vi "FTW-Reply-Construct.vi"(5 "Address":string, 11 "error in":errorcluster) -> (4 "FTW-Router Out":refnum<class "FTW-Reply.lvclass">, 6 "Actual Address":string, 10 "Event Registration Refnum":refnum<event-registration>, 15 "error out":errorcluster)   [LabVIEW 2013, in "FTW-Reply.lvclass"]
uses:
  FTW-Reply.lvclass
  Message/Request/FTW-Message-IncomingRequest.lvclass
  Ether/FTW-Ether-EndpointType.ctl
  Endpoint/FTW-Endpoint.lvclass
  FTW-Reply.lvclass/FTW-Reply.ctl
  Ether/FTW-Ether.lvclass
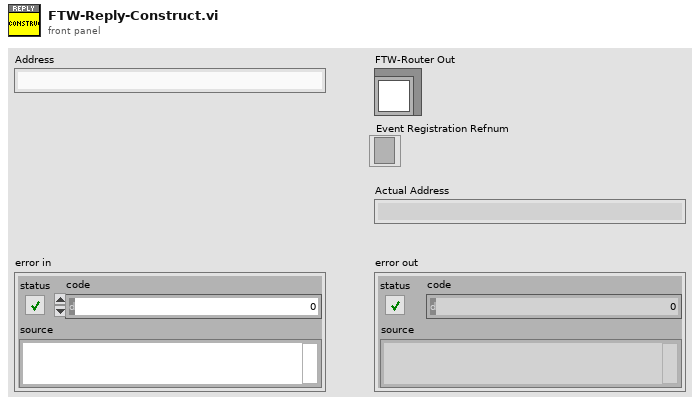
[diagram p1: front panel]
types:
  T1 = typedef "FTW-Ether.lvclass/FTW-Ether-EndpointType.ctl" = enum16{"Server", "Client", "Publisher", "Subscriber"}
  T2 = typedef "FTW-Ether.lvclass/FTW-Ether-MessageTransportScheme.ctl" = enum16{"In process (inproc://)", "TCP (tcp://)"}
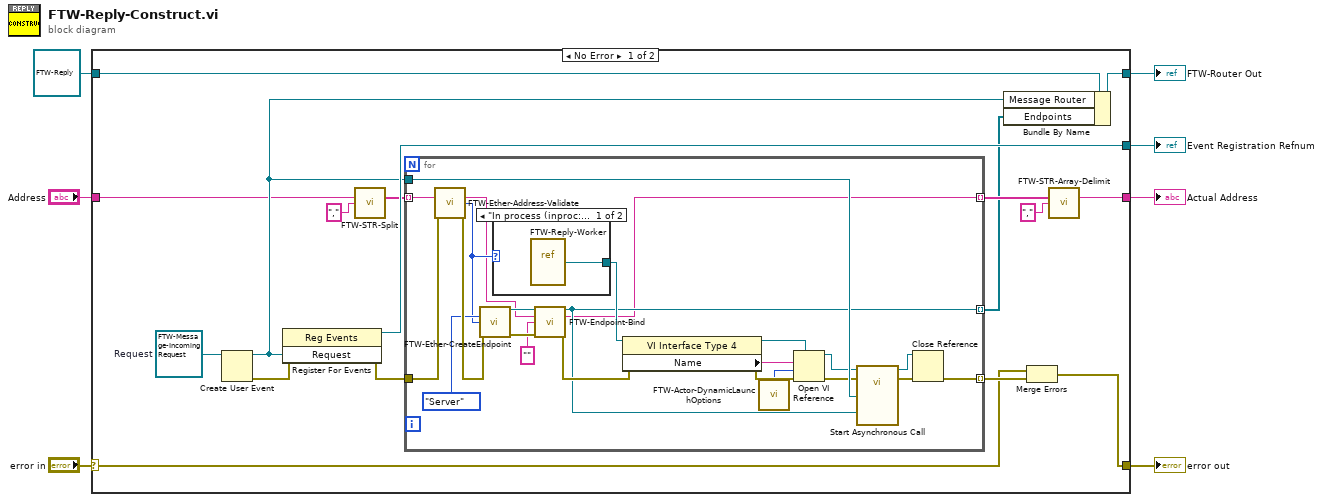
[diagram p0: block diagram]
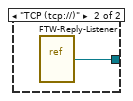
[diagram p2: hidden frame]
diagram:
  n1 = case shown="No Error" "error in" {
    selector: "error in" -> [w9 w51]
    tunnel: [w11 w51] -> w6
    tunnel: [w24 w50] -> w5
    tunnel: [w23 _] -> w3
    tunnel: "Address" -> [w15 _]
    tunnel: [w13 _] -> w2
    tunnel: refnum<class "FTW-Reply.lvclass"> refnum ("LVmsg_Router.lvclass") -> [w19 w50]
    frame No Error {
      w22 = refnum<class "FTW-Message-IncomingRequest.lvclass"> refnum  # Request
      n2 = Create User Event(user event datatype=w22) -> (user event=w20:refnum<user-event>, error out=w17:errorcluster)  [unwired: 1 in]
      n3 = register-events(error in=w17, w20) -> (reference out=w23:refnum<event-registration>, error out=w10:errorcluster)  [unwired: 1 in]
      n4 = call "FTW-STR-Split.vi"("Delimited String"=w15, "Delimiter"=",") -> ("Array of Strings"=w8:string[])  [unwired: 13 in]
      n5 = for {
        tunnel: [w25] -> w21 mode=indexing
        tunnel: w20 -> [w46]
        tunnel: w10 -> [w44]
        tunnel: [w43] -> w18 mode=indexing
        tunnel: w8 -> [w42] mode=indexing
        tunnel: [w28] -> w14 mode=indexing
        n6 = call "FTW-Ether-Address-Validate.vi"("Address"=w42, "error in"=w44) -> ("Sanitized Address"=w26:string, "Message Transport Scheme"=w31:T2, "error out"=w47:errorcluster)  [unwired: 11 in]
        n7 = call "FTW-Ether-CreateEndpoint.vi"("Endpoint Type"=FTW-Ether-EndpointType."Server", "Message Transport Scheme"=w31, "error in"=w47) -> ("FTW Endpoint"=w29:refnum<class "FTW-Endpoint.lvclass">, "error out"=w45:errorcluster)  [unwired: 11 in]
        n8 = case shown="\"In process (inproc://)\"" w31 {
          tunnel: [w48 w49] -> w40
          frame "In process (inproc://)" {
            n9 = vi-ref "FTW-Reply-Worker.vi"() -> (w48:refnum<vi>)
          }
          frame "TCP (tcp://)" {
            n10 = vi-ref "FTW-Reply-Listener.vi"() -> (w49:refnum<vi>)
          }
        }
        n11 = call-dynamic "FTW-Endpoint-Bind.vi"("FTW Endpoint"=w29, "Endpoint Address"=w26, "Requested Identity"="", "error in"=w45) -> ("FTW Endpoint out"=w28:refnum<class "FTW-Endpoint.lvclass">, "Actual Endpoint Address"=w25:string, "error out"=w30:errorcluster)  [unwired: 8 in, 1 out]
        n12 = property class="VI Interface Type 4"(reference=w40, error in=w30) -> (reference out=w36:refnum<vi>, error out=w39:errorcluster, "Name"=w38:string)
        n13 = call "FTW-Actor-DynamicLaunchOptions.vi"() -> ("Open VI Ref Options"=w37:i32)
        n14 = Open VI Reference(type specifier VI Refnum (for type only)=w36, vi path=w38, options=w37, error in (no error)=w39) -> (vi reference=w34:refnum<vi>, error out=w32:errorcluster)  [unwired: 2 in]
        n15 = call-by-ref "Start Asynchronous Call"(reference=w34, error in=w32, "Endpoint"=w28, "Message Handler"=w46) -> (reference out=w33:refnum<vi>, error out=w35:errorcluster)  [unwired: 1 in]
        n16 = Close Reference(reference=w33, error in (no error)=w35) -> (error out=w43:errorcluster)
      }
      n17 = Bundle By Name(cluster=w19, "Message Router"=w20, "Endpoints"=w14) -> (w24:refnum<class "FTW-Reply.lvclass">)
      n18 = Merge Errors(w9, w18) -> (w11:errorcluster)
      n19 = call "FTW-STR-Array-Delimit.vi"("Array of Strings"=w21, "Delimiter"=",") -> ("Delimited String"=w13:string)  [unwired: 13 in]
    }
    frame Error {
    }
  }
  "FTW-Router Out" <- w5
  "error out" <- w6
  "Event Registration Refnum" <- w3
  "Actual Address" <- w2
